vi "PolynomialFeatures.vi"(8 "error in (no error)":errorcluster caption="entrée d'erreur (pas d'erreur)", 11 "PolynomialFeatures":T1={"degre"=2, "interaction_only"=FALSE, "include_bias"=TRUE, "order"="C"}) -> (0 "error out":errorcluster, 3 "PolynomialFeatures.lvclass":refnum<class "PolynomialFeatures.lvclass">)   [LabVIEW 2020]
doc: "Generate polynomial and interaction features.\n\nGenerate a new feature matrix consisting of all polynomial combinations of the features with degree less than or equal to the specified degree. For example, if an input sample is two dimensional and of the form [a, b], the degree-2 polynomial features are [1, a, b, a^2, ab, b^2].\n\n\nParameters : \n\n- degree : integer\nThe degree of the polynomial features. Default = 2.\n\n- interaction_only : boolean, default = False\nIf true, only interaction features are produced: features that are products of at most degree distinct input features (so not x[1] ** 2, x[0] * x[2] ** 3, etc.).\n\n- include_bias : boolean\nIf True (default), then include a bias column, the feature in which all polynomial powers are zero (i.e. a column of ones - acts as an intercept term in a linear model).\n\n- order : str in {‘C’, ‘F’}, default ‘C’\nOrder of output array in the dense case. ‘F’ order is faster to compute, but may slow down subsequent estimators.\n\n\nMethods : \n\n\n- Fit : Compute number of output features.\n\nParameters : X : array-like, shape (n_samples, n_features)\n The data.\n\n- Fit Transform : Fit to data, then transform it. Fits transformer to X and y with optional parameters fit_params and returns a transformed version of X.\n\nParameters : X : {array-like, sparse matrix, dataframe} of shape (n_samples, n_features)\n y : ndarray of shape (n_samples,), default=None\n Target values.\n\nReturns : X_new : ndarray array of shape (n_samples, n_features_new)\n Transformed array.\n\n\n- Feature Names : Return feature names for output features\n\nReturns : output_feature_names : list of string, length n_output_features\n\n\n- Transform : Transform data to polynomial features\n\nParameters : \n\nX : array-like or CSR/CSC sparse matrix, shape [n_samples, n_features]\nThe data to transform, row by row.\n\nPrefer CSR over CSC for sparse input (for speed), but CSC is required if the degree is 4 or higher. If the degree is less than 4 and the input format is CSC, it will be converted to CSR, have its polynomial features generated, then converted back to CSC.\n\nIf the degree is 2 or 3, the method described in “Leveraging Sparsity to Speed Up Polynomial Feature Expansions of CSR Matrices Using K-Simplex Numbers” by Andrew Nystrom and John Hughes is used, which is much faster than the method used on CSC input. For this reason, a CSC input will be converted to CSR, and the output will be converted back to CSC prior to being returned, hence the preference of CSR.\n\nReturns : \n\nX : Pnp.ndarray or CSR/CSC sparse matrix, shape [n_samples, NP]\nThe matrix of features, where NP is the number of polynomial features generated from the combination of inputs."
uses:
  PolynomialFeatures.lvclass
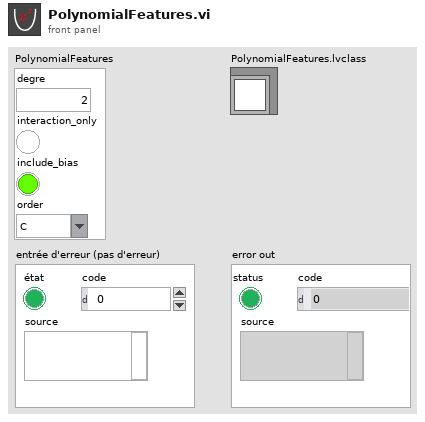
[diagram p1: front panel]
types:
  T1 = cluster{"degre":i32, "interaction_only":bool, "include_bias":bool, "order":string}
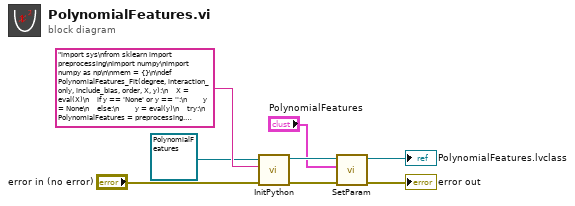
[diagram p0: block diagram]
diagram:
  n1 = call-dynamic "InitPython.vi"("error in (no error)"="error in (no error)", "Python Instruction"="import sys\nfrom sklearn import preprocessing\nimport numpy\nimport numpy as np\n\nmem = {}\n\ndef PolynomialFeatures_Fit(degree, interaction_only, include_bias, order, X, y):\n    X = eval(X)\n    if y == 'None' or y == '':\n        y = None\n    else:\n        y = eval(y)\n    try:\n        PolynomialFeatures = preprocessing.PolynomialFeatures(degree, interaction_only, include_bias, order).fit(X, y)\n        mem['FitPolynomialFeatures'] = PolynomialFeatures\n        return str('OK')\n    except:\n        erreur = sys.exc_info()\n        typerr = u\"%s\" % (erreur[0])\n        typerr = typerr[typerr.find(\"'\")+1:typerr.rfind(\"'\")]\n        msgerr = u\"%s\" % (erreur[1])\n        message = str('/!\\\\ {0} : {1}'. format(typerr,msgerr))\n        return message \n    \ndef PolynomialFeatures_FitTransform(degree, interaction_only, include_bias, order, X, y):\n    X = eval(X)\n    if y == 'None' or y == '':\n        y = None\n    else:\n        y = eval(y)\n    try:\n        PolynomialFeatures = preprocessing.PolynomialFeatures(degree, interaction_only, include_bias, order).fit_transform(X, y)\n        dtype = type(PolynomialFeatures)\n        if dtype == numpy.ndarray:\n            PolynomialFeatures = PolynomialFeatures.tolist()\n            return str(PolynomialFeatures) \n        else:\n            Mat = PolynomialFeatures.tocoo()\n            return str(list(zip(Mat.row, Mat.col, Mat.data)))\n    except:\n        erreur = sys.exc_info()\n        typerr = u\"%s\" % (erreur[0])\n        typerr = typerr[typerr.find(\"'\")+1:typerr.rfind(\"'\")]\n        msgerr = u\"%s\" % (erreur[1])\n        message = str('/!\\\\ {0} : {1}'. format(typerr,msgerr))\n        return message \n\ndef PolynomialFeatures_Transform(degree, interaction_only, include_bias, order, X, y):\n    X = eval(X)\n    if y == 'None' or y == '':\n        y = None\n    else:\n        y = eval(y)\n    try:\n        PolynomialFeatures = mem['FitPolynomialFeatures'].transform(X)\n        dtype = type(PolynomialFeatures)\n        if dtype == numpy.ndarray:\n            PolynomialFeatures = PolynomialFeatures.tolist()\n            return str(PolynomialFeatures) \n        else:\n            Mat = PolynomialFeatures.tocoo()\n            return str(list(zip(Mat.row, Mat.col, Mat.data)))\n    except:\n        erreur = sys.exc_info()\n        typerr = u\"%s\" % (erreur[0])\n        typerr = typerr[typerr.find(\"'\")+1:typerr.rfind(\"'\")]\n        msgerr = u\"%s\" % (erreur[1])\n        message = str('/!\\\\ {0} : {1}'. format(typerr,msgerr))\n        return message\n    \ndef PolynomialFeatures_Feature_Names(degree, interaction_only, include_bias, order, X):\n    try:\n        PolynomialFeatures = mem['FitPolynomialFeatures'].get_feature_names()\n        return str(PolynomialFeatures)\n    except:\n        erreur = sys.exc_info()\n        typerr = u\"%s\" % (erreur[0])\n        typerr = typerr[typerr.find(\"'\")+1:typerr.rfind(\"'\")]\n        msgerr = u\"%s\" % (erreur[1])\n        message = str('/!\\\\ {0} : {1}'. format(typerr,msgerr))\n        return message", "Scikit-learn en entrée"=refnum<class "PolynomialFeatures.lvclass"> refnum ("PolynomialFeatures.lvclass")) -> ("error out"=w4:errorcluster, "Scikit-learn en sortie"=w5:refnum<class "PolynomialFeatures.lvclass">)  [unwired: 7 in]
  n2 = call-dynamic "SetParam.vi"("error in (no error)"=w4, "PolynomialFeatures"="PolynomialFeatures", "PolynomialFeatures.lvclass"=w5) -> ("error out"=→"error out":errorcluster, "PolynomialFeatures.lvclass"=→"PolynomialFeatures.lvclass":refnum<class "PolynomialFeatures.lvclass">)  [unwired: 7 in]
